vi "Prepocty FINAL.vi"(3 "Ui":dbl[](array[numeric]), 4 "Uh":dbl[](array[numeric]), 5 "dt":dbl=1.0, 6 "N2":dbl=20.0, 7 "N1":dbl=131.0, 8 "h":dbl=0.005, 9 "r2":dbl=0.0125, 10 "r1":dbl=0.01, 11 "Rn":dbl=4.7) -> (0 "I":dbl[](array[numeric]), 1 "B":dbl[](array[numeric]), 2 "H":dbl[](array[numeric]))   [LabVIEW 2018]
uses:
  <vilib>/Analysis/2dsp.llb/Integral Method.ctl
  <vilib>/Analysis/baseanly.llb/Mean (DBL).vi
  <vilib>/Analysis/NI_AALPro.lvlib
  <vilib>/Analysis/NI_AALBase.lvlib
panel:
  out "x*y 2":dbl
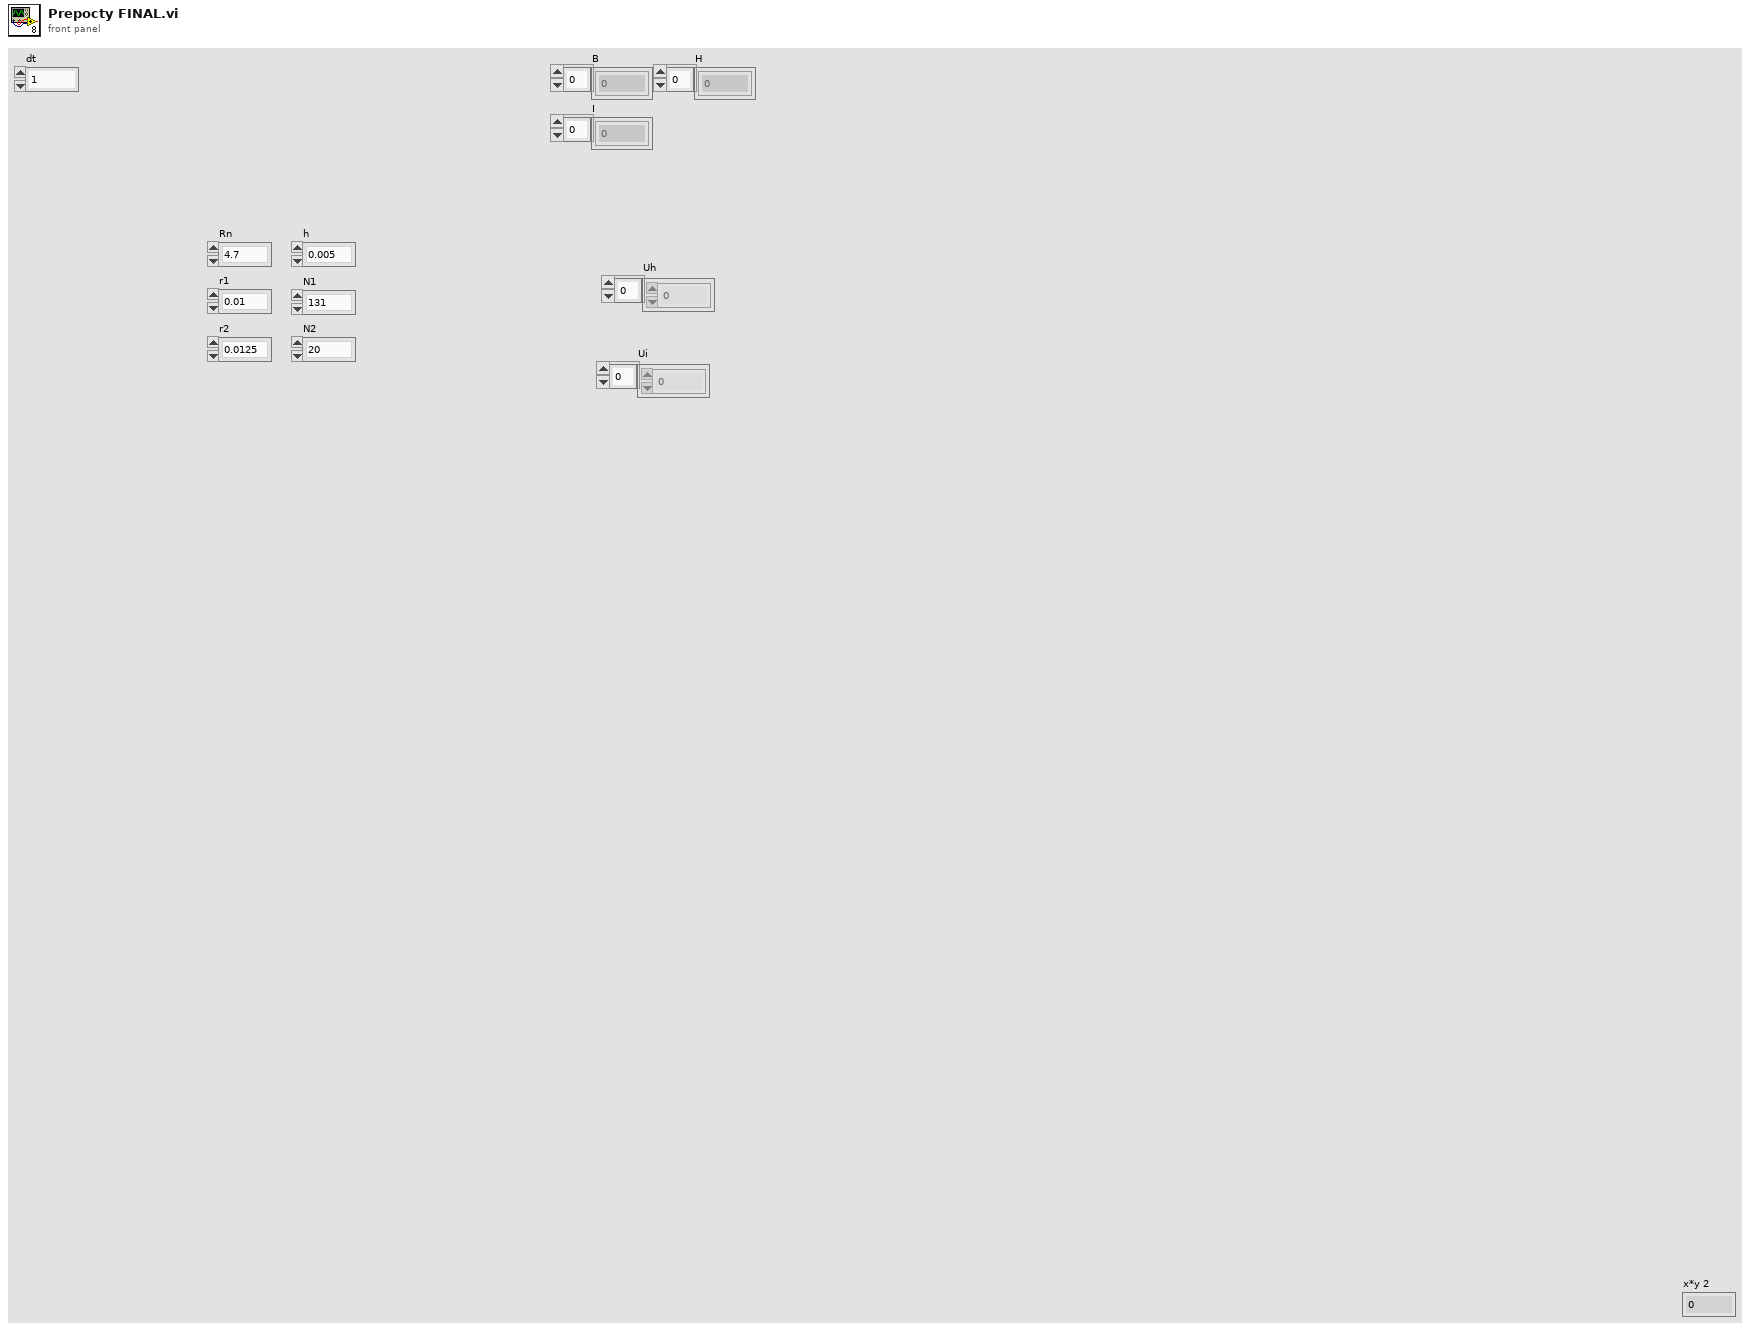
[diagram p1: front panel]
types:
  T1 = typedef "NI_AALPro.lvlib/Integral Method.ctl" = i32
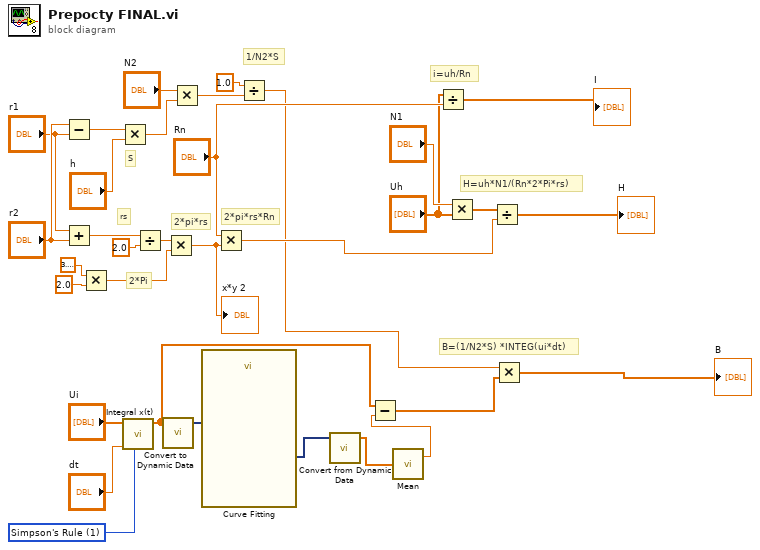
[diagram p0: block diagram]
diagram:
  w10 = T1 1 items=["Trapezoidal Rule", "Simpson's Rule", "Simpson's 3/8 Rule", "Bode Rule"] ("integration method")
  # "B=(1/N2*S) *INTEG(ui*dt)"
  # "1/N2*S"
  # "i=uh/Rn"
  # "2*pi*rs*Rn"
  # "2*pi*rs"
  # "2*Pi"
  # "H=uh*N1/(Rn*2*Pi*rs)"
  # "S"
  # "rs"
  n1 = Subtract(x="r2", y="r1") -> (x-y=w29:dbl)
  n2 = Add(x="r1", y="r2") -> (x+y=w33:dbl)
  n3 = Multiply(x=3.141592653589793, y=2.0) -> (x*y=w22:dbl)
  n4 = Multiply(x=w29, y="h") -> (x*y=w18:dbl)
  n5 = call <vilib>:"Integral x(t).vi"("integration method"=w10, "dt"="dt", "X"="Ui") -> ("Integral X"=w9:dbl[])  [unwired: 7 in, 1 out]
  n6 = Divide(x=w33, y=2.0) -> (x/y=w25:dbl)
  n7 = call "Convert to Dynamic Data"("Array"=w9) -> ("Dynamic Data Type"=w12:dynamicdata)  [unwired: 3 in]
  n8 = Multiply(x=w25, y=w22) -> (x*y=w21:dbl)
  "x*y 2" <- w21
  n9 = Multiply(x="N2", y=w18) -> (x*y=w17:dbl)
  n10 = call "Curve Fitting"("Signals"=w12) -> ("best fit"=w8:dynamicdata)  [unwired: 6 in, 4 out]
  n11 = Multiply(x="Rn", y=w21) -> (x*y=w20:dbl)
  n12 = Divide(x=1.0, y=w17) -> (x/y=w7:dbl)
  n13 = call "Convert from Dynamic Data"("Dynamic Data Type"=w8) -> ("Array"=w2:dbl[])  [unwired: 3 in]
  n14 = call-poly <vilib>:"Mean.vi"("X"=w2) -> ("mean"=w1:dbl)  [unwired: 1 out]
  n15 = Subtract(x=w9, y=w1) -> (x-y=w6:dbl[])
  n16 = Divide(x="Uh", y="Rn") -> (x/y=→"I":dbl[])
  n17 = Multiply(x="N1", y="Uh") -> (x*y=w26:dbl[])
  n18 = Divide(x=w26, y=w20) -> (x/y=→"H":dbl[])
  n19 = Multiply(x=w7, y=w6) -> (x*y=→"B":dbl[])
